vi "Get Sciscan Scope Image Refresh.vi"(8 "error in":errorcluster, 11 "GFG Refnum":refnum<vi>) -> (0 "error out":errorcluster, 2 "display every n-th frame":i8=10, 3 "GFG Refnum Out":refnum<vi>)   [LabVIEW 2012, in "Sciscan Scope Daemon.lvlib"]
uses:
  Sciscan Scope Daemon.lvlib
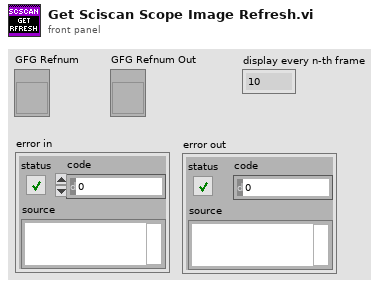
[diagram p1: front panel]
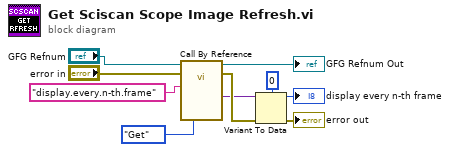
[diagram p0: block diagram]
diagram:
  n1 = call-by-ref "?"(reference="GFG Refnum", error in="error in", "Variable Name in"="display.every.n-th.frame", "Action"=enum16{"Init", "Set", "Get"}."Get") -> (reference out=→"GFG Refnum Out":refnum<vi>, error out=w6:errorcluster, "Variant Out"=w5:variant)  [unwired: 11 in, 6 out]
  n2 = Variant To Data(error in=w6, type=i8 0 ("display every n-th frame"), Variant=w5) -> (data=→"display every n-th frame":i8, error out=→"error out":errorcluster)
